vi "SQL_test_template_update.vi"(11 "表格控件":string[][](table)) -> (3 "error out":errorcluster)   [LabVIEW 2014]
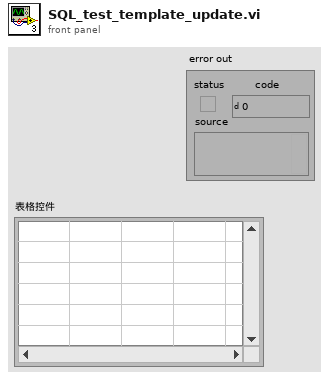
[diagram p1: front panel]
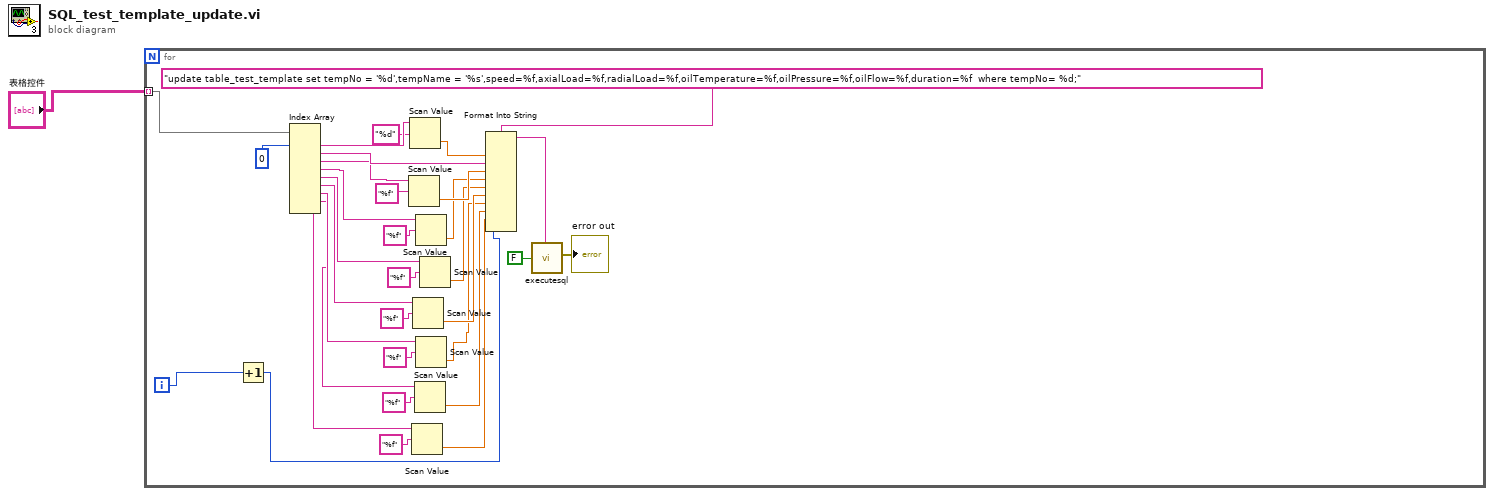
[diagram p0: block diagram]
diagram:
  n1 = for {
    tunnel: "表格控件" -> [w30] mode=indexing
    i -> [w27]
    n2 = Increment(x=w27) -> (x+1=w3:i32)
    n3 = Index Array(array=w30, index #1=0 ("索引")) -> (element #1=w14:string, element #2=w26:string, element #3=w25:string, element #4=w22:string, element #5=w19:string, element #6=w17:string, element #7=w11:string, element #8=w7:string, element #9=w4:string)  [unwired: 8 in]
    n4 = Scan Value(string=w25, format string="%f" ("格式字符串")) -> (value=w24:dbl)  [unwired: 1 in, 1 out]
    n5 = Scan Value(string=w14, format string="%d") -> (value=w15:dbl)  [unwired: 1 in, 1 out]
    n6 = Scan Value(string=w4, format string="%f" ("格式字符串")) -> (value=w5:dbl)  [unwired: 1 in, 1 out]
    n7 = Scan Value(string=w17, format string="%f" ("格式字符串")) -> (value=w16:dbl)  [unwired: 1 in, 1 out]
    n8 = Scan Value(string=w7, format string="%f" ("格式字符串")) -> (value=w8:dbl)  [unwired: 1 in, 1 out]
    n9 = Scan Value(string=w22, format string="%f" ("格式字符串")) -> (value=w23:dbl)  [unwired: 1 in, 1 out]
    n10 = Scan Value(string=w11, format string="%f" ("格式字符串")) -> (value=w10:dbl)  [unwired: 1 in, 1 out]
    n11 = Scan Value(string=w19, format string="%f" ("格式字符串")) -> (value=w18:dbl)  [unwired: 1 in, 1 out]
    n12 = Format Into String(format string="update table_test_template set tempNo = '%d',tempName = '%s',speed=%f,axialLoad=%f,radialLoad=%f,oilTemperature=%f,oilPressure=%f,oilFlow=%f,duration=%f  where tempNo= %d;", w15, w26, w24, w23, w18, w16, w10, w8, w5, w3) -> (resulting string=w32:string)  [unwired: 2 in, 1 out]
    n13 = call "executesql.vi"("Return Data (T)"=FALSE, "Command Text"=w32) -> ("error out"=→"error out":errorcluster)  [unwired: 5 in, 1 out]
  }
